vi "SaveFalconImage.vi"(0 "SavePath":path, 1 "Binning":u16, 2 "ROIYOffset":u16, 3 "ROIXOffset":u16, 4 "PixScale1":dbl=2008.731741 format="%.2f", 7 "Image":u16[][](array[numeric]), 11 "EXPTIME":dbl, 12 "RA Sonde":dbl=70407.2665759738 caption="RA de la sonde" format="%<%H:%M:%S%1u>t", 13 "Dec Sonde":dbl=34150.89703708518 caption="DEC de la sonde" format="%<%H:%M:%S%0u>t", 14 "Epoch Tel":dbl=2008.731741 caption="Époque" format="%.2f", 15 "PixScale2":dbl=2008.731741 format="%.2f") -> ()   [LabVIEW 2011]
uses:
  gfitsio/cfitsio-bitpix.ctl
  fits/AddHeaderParams(INT).vi
  fits/AddHeaderParams(STR).vi
  fits/AddHeaderParams(DBL).vi
  gfitsio/gfitsio.lvlib
panel:
  out "error out":errorcluster
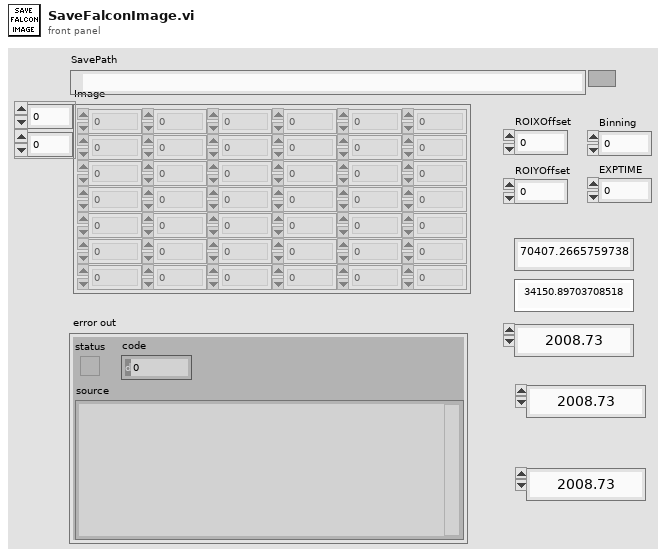
[diagram p1: front panel]
types:
  T1 = typedef "gfitsio.lvlib/cfitsio-bitpix.ctl" = i32
  T2 = enum16{"open", "open or create", "create", "create or replace"}
  T3 = enum16{"open", "open or create", "create or replace", "create", "open (read only)"}
  T4 = cluster{"comment":string, i32, "comment":string, "units":string}
  T5 = typedef "gfitsio.lvlib/gfitsio-refnum.ctl" = refnum<k1>
  T6 = cluster{"comment":string, "formatted-str":string, "comment":string, "units":string}
  T7 = cluster{"comment":string, "Epoch Tel":dbl, "comment":string, "units":string}
  T8 = cluster{"comment":string, dbl, "comment":string, "units":string}
  T9 = cluster{"comment":string, "formatted-str":string, "comment":string, "units":string}[]
  T10 = cluster{"comment":string, i32, "comment":string, "units":string}[]
  T11 = cluster{"comment":string, "Epoch Tel":dbl, "comment":string, "units":string}[]
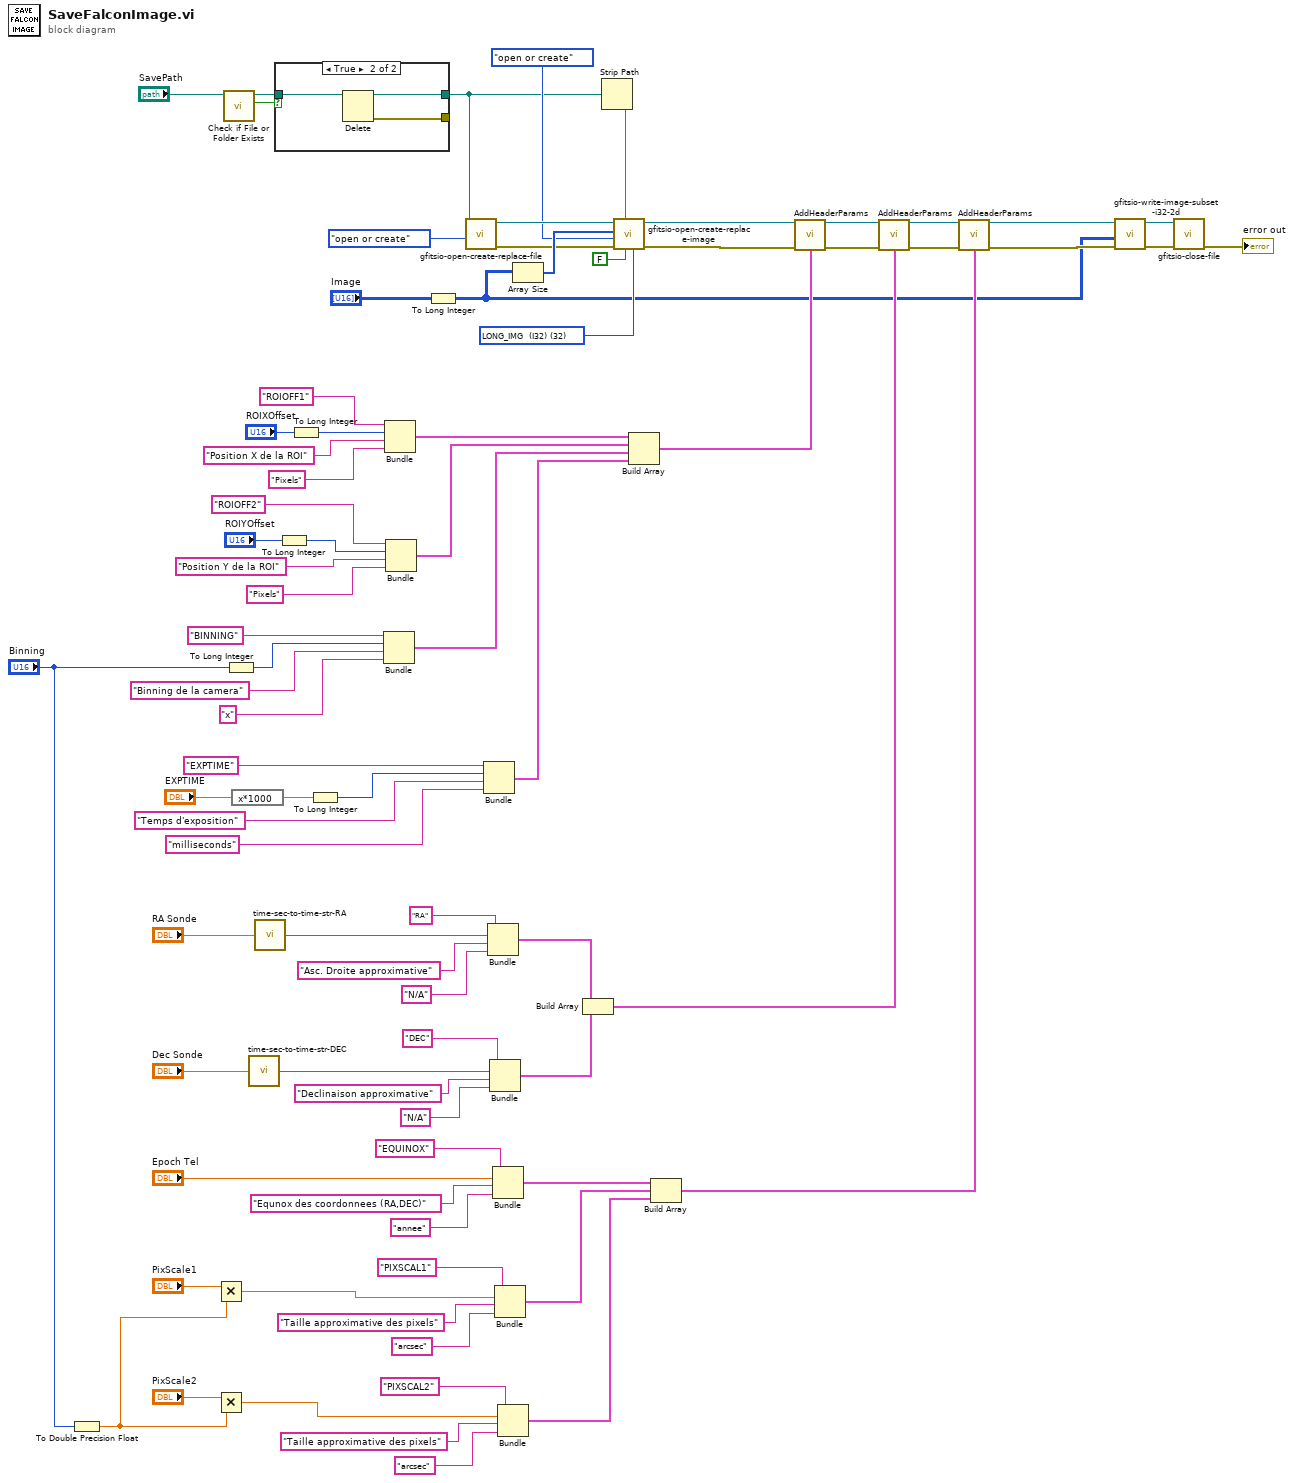
[diagram p0: block diagram]
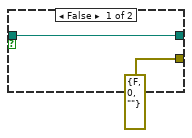
[diagram p2: hidden frame]
diagram:
  w76 = T1 32 items=["<invalid type>"=0, "BYTE_IMG  (U8)"=8, "SHORT_IMG  (I16)"=16, "USHORT_IMG  (U16)"=20, "LONG_IMG  (I32)"=32, "ULONG_IMG  (U32)"=40, "FLOAT_IMG  (SGL)"=-32, "DOUBLE_IMG  (DBL)"=-64] ("image data type")
  n1 = To Double Precision Float(number="Binning") -> (double precision float=w4:dbl)
  n2 = Multiply(x="PixScale1", y=w4) -> (x*y=w1:dbl)
  n3 = Multiply(x="PixScale2", y=w4) -> (x*y=w2:dbl)
  n4 = call <vilib>:"Check if File or Folder Exists.vi"("path"="SavePath") -> ("file or folder exists?"=w73:bool, "dup path"=w72:path)  [unwired: 8 in, 1 out]
  n5 = To Long Integer(number="Binning") -> (32bit integer=w51:i32)
  n6 = expression code="x*1000"("EXPTIME") -> (w41:dbl)
  n7 = call "time-sec-to-time-str-DEC.vi"("Numeric"="Dec Sonde") -> ("formatted-str"=w38:string)
  n8 = call "time-sec-to-time-str-RA.vi"("Numeric"="RA Sonde") -> ("formatted-str"=w33:string)
  n9 = case shown="True" w73 {
    tunnel: w72 -> [w85 w88]
    tunnel: [w85 w87] -> w15
    tunnel: [errorcluster {"status"=FALSE, "code"=0, "source"=""} ("error out") w86] -> _
    frame False {
    }
    frame True {
      n10 = Delete(path (use dialog)=w88) -> (deleted path=w87:path, error out=w86:errorcluster)  [unwired: 4 in, 1 out]
    }
  }
  n11 = To Long Integer(number="ROIYOffset") -> (32bit integer=w59:i32)
  n12 = To Long Integer(number="ROIXOffset") -> (32bit integer=w64:i32)
  n13 = To Long Integer(number=w41) -> (32bit integer=w47:i32)
  n14 = Bundle("comment"="BINNING", w51, "comment"="Binning de la camera", "units"="x") -> (w52:T4)  [unwired: 1 in]
  n15 = Bundle("comment"="ROIOFF1", w64, "comment"="Position X de la ROI", "units"="Pixels") -> (w61:T4)  [unwired: 1 in]
  n16 = Bundle("comment"="ROIOFF2", w59, "comment"="Position Y de la ROI", "units"="Pixels") -> (w56:T4)  [unwired: 1 in]
  n17 = To Long Integer(number="Image") -> (32bit integer=w17:i32[][])
  n18 = call "gfitsio-open-create-replace-file.vi"("function (open)"=T3."open or create", "file path (dialog if empty)"=w15) -> ("error out"=w77:errorcluster, "gfits refnum"=w81:T5)  [unwired: 7 in, 1 out]
  n19 = Bundle("comment"="EXPTIME", w47, "comment"="Temps d'exposition", "units"="milliseconds") -> (w43:T4)  [unwired: 1 in]
  n20 = Bundle("comment"="RA", "formatted-str"=w33, "comment"="Asc. Droite approximative", "units"="N/A") -> (w30:T6)  [unwired: 1 in]
  n21 = Bundle("comment"="DEC", "formatted-str"=w38, "comment"="Declinaison approximative", "units"="N/A") -> (w29:T6)  [unwired: 1 in]
  n22 = Bundle("comment"="EQUINOX", "Epoch Tel"="Epoch Tel", "comment"="Equnox des coordonnees (RA,DEC)", "units"="annee") -> (w19:T7)  [unwired: 1 in]
  n23 = Bundle("comment"="PIXSCAL1", w1, "comment"="Taille approximative des pixels", "units"="arcsec") -> (w8:T8)  [unwired: 1 in]
  n24 = Bundle("comment"="PIXSCAL2", w2, "comment"="Taille approximative des pixels", "units"="arcsec") -> (w7:T8)  [unwired: 1 in]
  n25 = Array Size(array=w17) -> (size(s)=w83:i32[])
  n26 = Build Array(w30, w29) -> (w28:T9)
  n27 = Strip Path(path=w15) -> (name=w78:string)  [unwired: 1 out]
  n28 = call "gfitsio-open-create-replace-image.vi"("image data type"=w76, "advisory dialog? (display:T)"=FALSE, "hdu name (dialog if empty)"=w78, "error in (no error)"=w77, "function (open or create)"=T2."open or create", "naxes"=w83, "gfits refnum"=w81) -> ("error out"=w66:errorcluster, "dup gfits refnum"=w67:T5)  [unwired: 2 in, 1 out]
  n29 = Build Array(w61, w56, w52, w43) -> (w50:T10)
  n30 = Build Array(w19, w8, w7) -> (w18:T11)
  n31 = call-poly "AddHeaderParams.vi"("gfits refnum"=w67, "Error in"=w66, "IntegerLine"=w50) -> ("dup gfits refnum"=w49:T5, "Error out"=w48:errorcluster)  [unwired: 11 in]
  n32 = call-poly "AddHeaderParams.vi"("gfits refnum"=w49, "Error in"=w48, "IntegerLine"=w28) -> ("dup gfits refnum"=w27:T5, "Error out"=w26:errorcluster)  [unwired: 11 in]
  n33 = call-poly "AddHeaderParams.vi"("gfits refnum"=w27, "Error in"=w26, "IntegerLine"=w18) -> ("dup gfits refnum"=w25:T5, "Error out"=w24:errorcluster)  [unwired: 11 in]
  n34 = call "gfitsio-write-image-subset-i32-2d.vi"("error in (no error)"=w24, "data"=w17, "gfits refnum"=w25) -> ("error out"=w70:errorcluster, "dup gfits refnum"=w71:T5)  [unwired: 7 in]
  n35 = call "gfitsio-close-file.vi"("error in (no error)"=w70, "gfits refnum"=w71) -> ("error out"=→"error out":errorcluster)  [unwired: 8 in, 1 out]
